vi "FeedbackDecode_WriteTextEOL.vi"(8 "error in":errorcluster, 10 "text":string, 11 "refnum in":refnum<file>) -> (0 "error out":errorcluster, 3 "refnum out":refnum<file>)   [LabVIEW 2020]
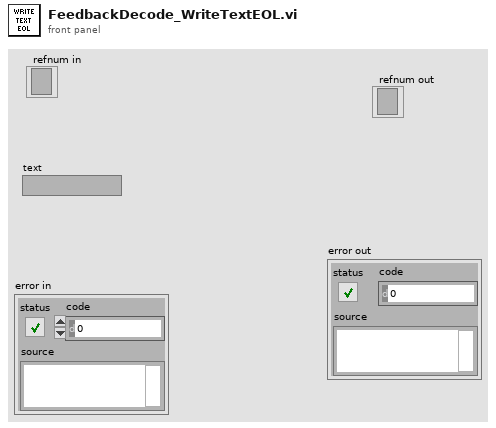
[diagram p1: front panel]
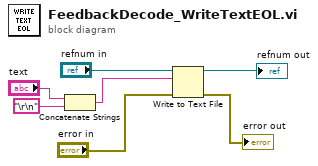
[diagram p0: block diagram]
diagram:
  n1 = Concatenate Strings("text", "\r\n") -> (w4:string)
  n2 = Write to Text File(file (use dialog)="refnum in", text=w4, error in="error in") -> (refnum out=→"refnum out":refnum<file>, error out=→"error out":errorcluster)  [unwired: 1 in, 1 out]
